vi "DeviceFacade.vi"(0 "Data In":T5={"device ID"=0, "Device Name"="", "number of samples/ch"=100000, "sample mode"=1, "sound format"={"sample rate (S/s)"=0.0, "number of channels"=2, "bits per sample"=16}, "Sample length (sec)"=0.5, "Pre-trigger (sec)"=0.1} {"Pre-trigger (sec)" min=0.0 max=32.0 step=0.1 format="%#_4f"; "Sample length (sec)" min=0.0 max=32.0 step=0.1 format="%#_4f"; "sample mode" items=["Finite Samples", "Continuous Samples"]}, 2 "Display State In":T3, 3 "Container State":T4) -> (6 "Data Out":T5={"device ID"=0, "Device Name"="", "number of samples/ch"=100000, "sample mode"=1, "sound format"={"sample rate (S/s)"=0.0, "number of channels"=2, "bits per sample"=16}, "Sample length (sec)"=0.5, "Pre-trigger (sec)"=0.1} {"Pre-trigger (sec)" min=0.0 max=32.0 step=0.1 format="%#_4f"; "Sample length (sec)" min=0.0 max=32.0 step=0.1 format="%#_4f"; "sample mode" items=["Finite Samples", "Continuous Samples"]}, 7 "Display State Out":T3, 8 "Action":T2)   [LabVIEW 2014, in "Audio Channel.xctl"]
uses:
  <userlib>/CurtinCode/Devicectrl/Audio Channel.xctl
  <userlib>/CurtinCode/Devicectrl/DeviceData.ctl
  <vilib>/sound2/lvsound2.llb/Sampling Mode.ctl
  <vilib>/sound2/lvsound2.llb/Sound Data Format.ctl
  <vilib>/_xctls/Container State.ctl
  <userlib>/CurtinCode/Devicectrl/DeviceState.ctl
  <vilib>/_xctls/Action.ctl
  <userlib>/CurtinCode/DAQType.ctl
  <vilib>/_xctls/XControlSupport.lvlib
panel:
  in  "Sample Trigger":dbl(slide)=0.1 scale=0.0..0.5
  in  "Headers":T1[](array[typedef]) items=["Hammer (V)", "Microphone (V)", "Accelerometer (g)"]
  in  "Refresh Button":bool
  in  "Sample rate (Hz)":dbl(slide)=44100.0 min=8000.0 max=48000.0 scale=8000.0..48000.0
  in  "#Channels":i32(ring)=2 items=["1"=1, "2"=2]
  in  "Resolution (bits)":i32=16 min=1 max=32
  in  "Device":u32(ring) items=["Microphone (High Definition Audio Device)"]
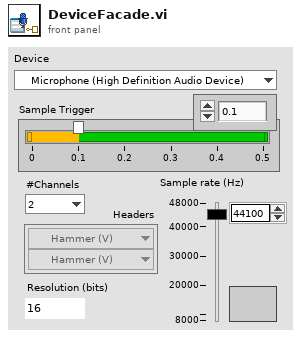
[diagram p1: front panel]
types:
  T1 = typedef "DAQType.ctl" = u16
  T2 = typedef "XControlSupport.lvlib/Action.ctl" = cluster{"Data Changed?":bool, "State Changed?":bool, "Action Name":string}
  T3 = typedef "Audio Channel.xctl/DeviceState.ctl" = cluster{"Numeric":dbl}
  T4 = typedef "XControlSupport.lvlib/Container State.ctl" = cluster{"Indicator?":bool, "Run Mode?":bool, " Refnum":refnum<vi>}
  T5 = typedef "Audio Channel.xctl/DeviceData.ctl" = cluster{"device ID":u32, "Device Name":string, "number of samples/ch":i32, "sample mode":T6, "sound format":T7, "Sample length (sec)":dbl, "Pre-trigger (sec)":dbl}
  T6 = typedef "Sampling Mode.ctl" = i32
  T7 = typedef "Sound Data Format.ctl" = cluster{"sample rate (S/s)":dbl, "number of channels":i32, "bits per sample":i32}
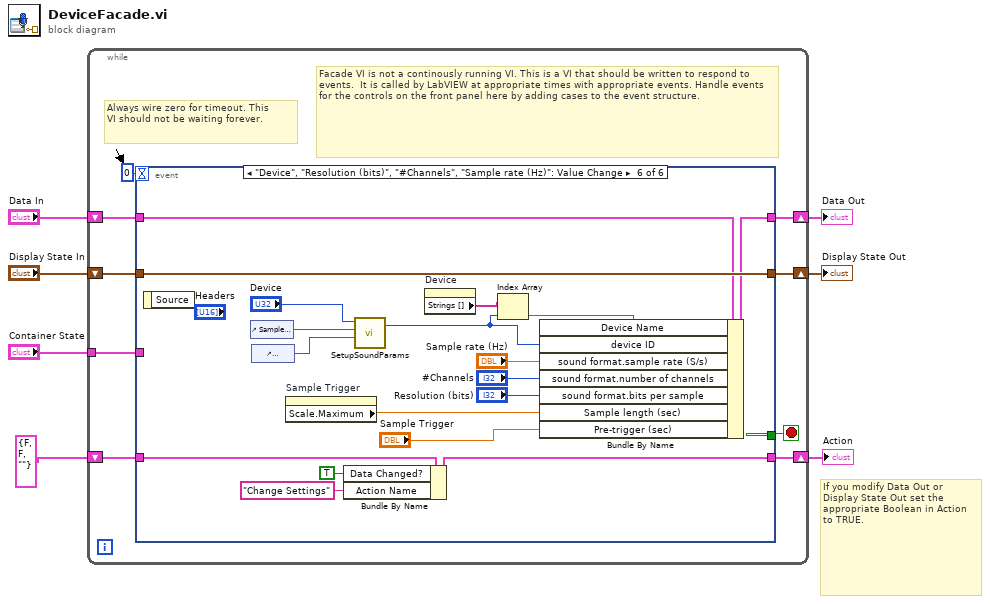
[diagram p0: block diagram]
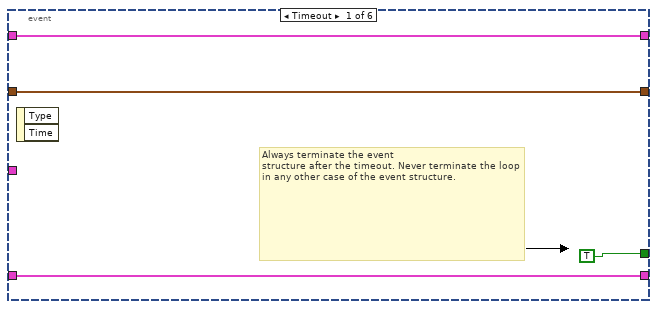
[diagram p2: hidden frame]
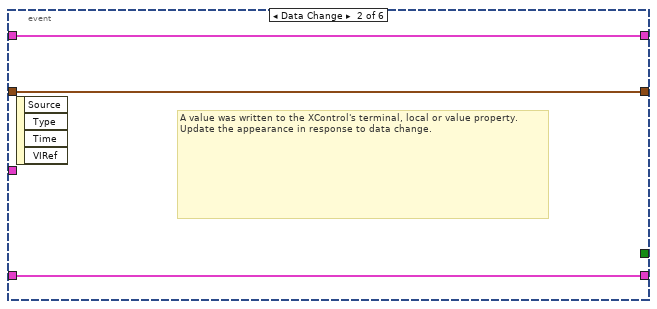
[diagram p3: hidden frame]
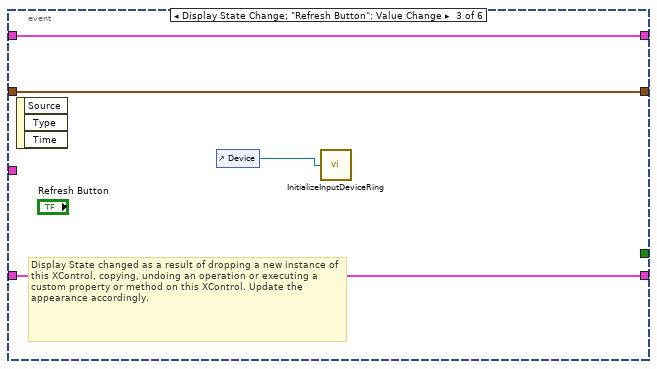
[diagram p4: hidden frame]
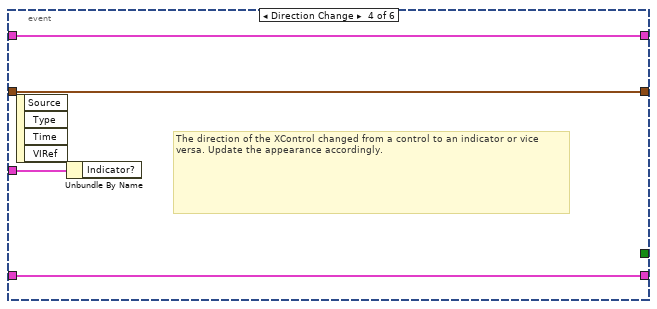
[diagram p5: hidden frame]
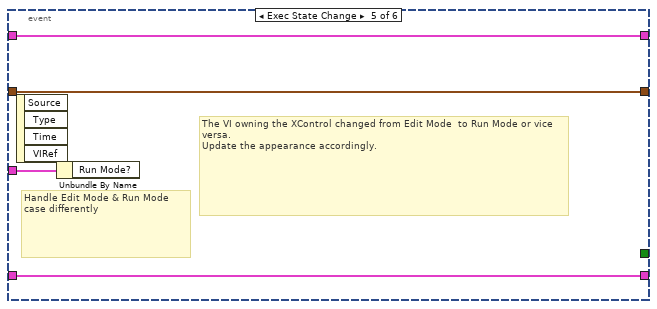
[diagram p6: hidden frame]
diagram:
  # "If you modify Data Out or\nDisplay State Out set the\nappropriate Boolean in Action\nto TRUE."
  n1 = while {
    shift-right: [w15] -> w4
    shift-left: "Display State In" -> [w16]
    tunnel: "Container State" -> [w12]
    shift-right: [w10] -> w7
    shift-left: "Data In" -> [w11]
    shift-right: [w8] -> w2
    shift-left: T2 {"Data Changed?"=FALSE, "State Changed?"=FALSE, "Action Name"=""} ("Action") -> [w9]
    stop <- w14 stop-if-true
    # "Facade VI is not a continously running VI. This is a VI that should be written to respond to events.  It is called by LabVIEW at appropriate times with appropriate events. Handle events for the controls on the front panel here by adding cases to the event structure."
    # "Always wire zero for timeout. This\nVI should not be waiting forever."
    n2 = event shown="[5] \"Device\", \"Resolution (bits)\", \"#Channels\", \"Sample rate (Hz)\": Value Change" {
      selector: _ -> [_ _ _ _ _ _]
      dyn-events: _ -> [_ _ _ _ _ _]
      timeout: 0 -> [_ _ _ _ _ _]
      tunnel: w16 -> [w18 w22 w27 w30 w34 w53]
      tunnel: [w18 w22 w27 w30 w34 w53] -> w15
      tunnel: [TRUE _ _ _ _ _] -> w14
      tunnel: w12 -> [_ _ _ w31 w35 _]
      tunnel: w11 -> [w17 w23 w26 w29 w33 w46]
      tunnel: [w17 w23 w26 w29 w33 w45] -> w10
      tunnel: [w19 w21 w25 w28 w32 w49] -> w8
      tunnel: w9 -> [w19 w21 w25 w28 w32 w52]
      event Timeout {
        # "Always terminate the event\nstructure after the timeout. Never terminate the loop in any other case of the event structure."
        n3 = event-data() -> ()  [unwired: 1 in, 2 out]
      }
      event Data Change {
        # "A value was written to the XControl's terminal, local or value property.\nUpdate the appearance in response to data change."
        n4 = event-data() -> ()  [unwired: 1 in, 4 out]
      }
      event Display State Change; "Refresh Button": Value Change {
        # "Display State changed as a result of dropping a new instance of this XControl, copying, undoing an operation or executing a custom property or method on this XControl. Update the appearance accordingly."
        n5 = event-data() -> ()  [unwired: 1 in, 3 out]
        n6 = control-ref of="Device"() -> (w24:refnum<vi>)
        n7 = call <vilib>:"InitializeInputDeviceRing.vi"("Device Refnum"=w24) -> ()  [unwired: 1 in, 14 out]
      }
      event Direction Change {
        # "The direction of the XControl changed from a control to an indicator or vice versa. Update the appearance accordingly."
        n8 = event-data() -> ()  [unwired: 1 in, 4 out]
        n9 = Unbundle By Name(w31) -> ()  [unwired: 1 out]
      }
      event Exec State Change {
        # "The VI owning the XControl changed from Edit Mode  to Run Mode or vice versa.\nUpdate the appearance accordingly."
        # "Handle Edit Mode & Run Mode\ncase differently"
        n10 = event-data() -> ()  [unwired: 1 in, 4 out]
        n11 = Unbundle By Name(w35) -> ()  [unwired: 1 out]
      }
      event "Device", "Resolution (bits)", "#Channels", "Sample rate (Hz)": Value Change {
        n12 = event-data() -> ()  [unwired: 1 in, 1 out]
        n13 = control-ref of="Sample rate (Hz)"() -> (w51:refnum<vi>)
        n14 = control-ref of="#Channels"() -> (w50:refnum<vi>)
        n15 = property on="Sample Trigger" class="Slide (strict)"() -> ("Scale.Maximum"=w36:dbl)  [unwired: 2 in, 2 out]
        n16 = Bundle By Name(cluster=w52, "Data Changed?"=TRUE, "Action Name"="Change Settings") -> (w49:T2)
        n17 = call <userlib>:"SetupSoundParams.vi"("#Channels"=w50, "Sample Rate (Hz)"=w51, "device"="Device") -> ("device out"=w39:u32)  [unwired: 1 in, 1 out]
        n18 = property on="Device" class="Ring (strict)"() -> ("Strings []"=w40:string[])  [unwired: 2 in, 2 out]
        n19 = Index Array(array=w40, index=w39) -> (element=w38:string)
        n20 = Bundle By Name(cluster=w46, "Device Name"=w38, "device ID"=w39, "sound format.sample rate (S/s)"="Sample rate (Hz)", "sound format.number of channels"="#Channels", "sound format.bits per sample"="Resolution (bits)", "Sample length (sec)"=w36, "Pre-trigger (sec)"="Sample Trigger") -> (w45:T5)
      }
    }
  }
  "Display State Out" <- w4
  "Data Out" <- w7
  "Action" <- w2
